vi "Read meas.oversample clock.vi"(11 "sync.resources":T1) -> (2 "meas.oversample clock":refnum<k21>, 3 "sync.resources":T1)   [LabVIEW 2014, in "ni579x Synchronization v2 FPGA.lvlib"]
uses:
  <instrlib>/ni579x/Synchronization/v2/FPGA/ni579x Synchronization v2 FPGA.lvlib
  <instrlib>/ni579x/Synchronization/v2/FPGA/Implementation/Resources.ctl
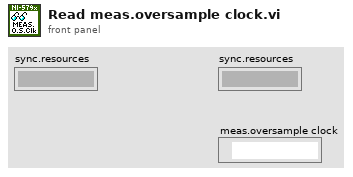
[diagram p1: front panel]
types:
  T1 = typedef "ni579x Synchronization v2 FPGA.lvlib/Resources.ctl" = cluster{"master":refnum<k21>, "meas.enable":refnum<k21>, "meas.ready":refnum<k21>, "meas.arm":refnum<k21>, "meas.valid":refnum<k21>, "meas.value":refnum<k21>, "meas.oversample clock":refnum<k21>, "meas.oversample factor":refnum<k21>, "cptr":refnum<k21>, "cptr.adjust":refnum<k21>, "cptr.period":refnum<k21>}
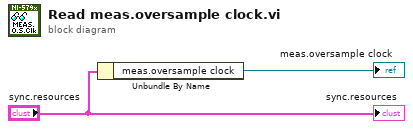
[diagram p0: block diagram]
diagram:
  n1 = Unbundle By Name("sync.resources") -> ("meas.oversample clock"=→"meas.oversample clock":refnum<k21>)
  "sync.resources" <- "sync.resources"
